vi "initDetection.vi"(8 "error in (no error)":errorcluster, 10 "detectionParameters":T1, 11 "dl in":refnum<class "dl.lvclass">) -> (0 "error out":errorcluster, 3 "dl out":refnum<class "dl.lvclass">)   [LabVIEW 2025, in "dl.lvlib" / "dl.lvclass"]
uses:
  dl.lvclass
  dl.lvclass/dl.ctl
  detectionParameters.ctl
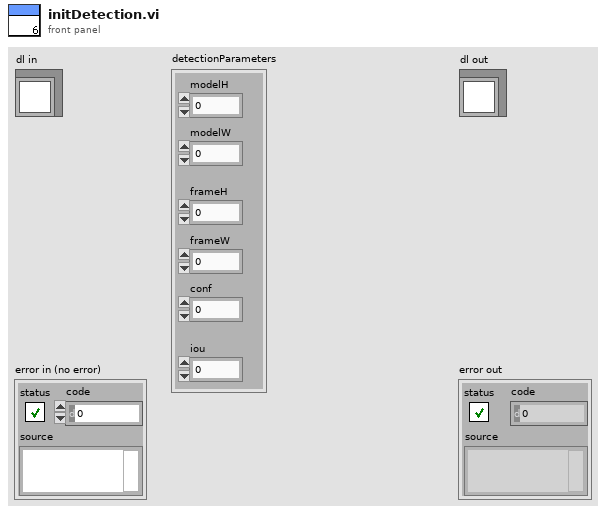
[diagram p1: front panel]
types:
  T1 = typedef "detectionParameters.ctl" = cluster{"modelH":i32, "modelW":i32, "frameH":i32, "frameW":i32, "conf":sgl, "iou":sgl}
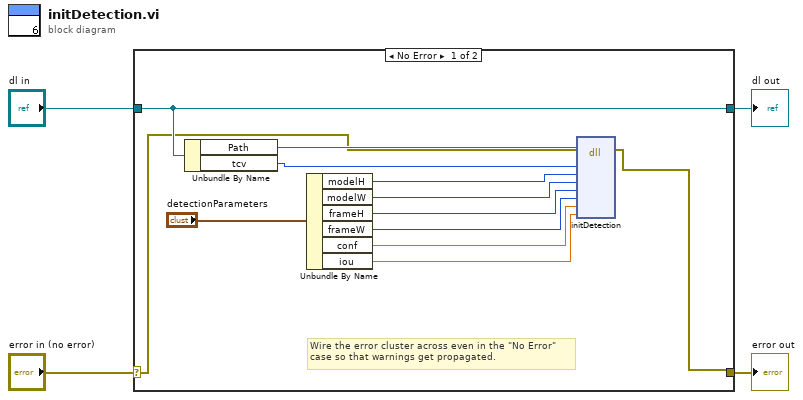
[diagram p0: block diagram]
diagram:
  n1 = case shown="No Error" "error in (no error)" {
    selector: "error in (no error)" -> [w13 w18]
    tunnel: [w12 w18] -> w3
    tunnel: [w16 w17] -> w1
    tunnel: "dl in" -> [w16 w17]
    frame No Error {
      # "Wire the error cluster across even in the \"No Error\"\ncase so that warnings get propagated."
      n2 = Unbundle By Name(w16) -> ("Path"=w15:path, "tcv"=w14:u64)
      n3 = Unbundle By Name("detectionParameters") -> ("modelH"=w10:i32, "modelW"=w9:i32, "frameH"=w8:i32, "frameW"=w7:i32, "conf"=w6:sgl, "iou"=w5:sgl)
      n4 = dll-call lib="D:/Test/adslvPackageDev/Resources/TCV_Lib.dll" fn="initDetection"(path in=w15, error in=w13, "tcv"=w14, "modelH"=w10, "modelW"=w9, "frameH"=w8, "frameW"=w7, "conf"=w6, "iou"=w5) -> (error out=w12:errorcluster)  [unwired: 9 in, 1 out]
    }
    frame Error {
    }
  }
  "error out" <- w3
  "dl out" <- w1
